vi "Charging_Extract Temp Thresholds From String.vi"(11 "Gen Cals In":string="Reserved[00]=0x00\nReserved[01]=0x00\nReserved[02]=0x00\nReserved[03]=0x00\nReserved[04]=0x00\nReserved[05]=0x00\nReserved[06]=0x00\nReserved[07]=0x00\nReserved[08]=0x00\t\t\nReserved[09]=0x00\nReserved[10]=0x00\nReserved[11]=0x00\nReserved[12]=0x00\nReserved[13]=0x00\nReserved[14]=0x00\ntempMinThreshold=0xCAC4\ntempWarningThresholdl=0x31D3\ntempCriticalThresholdl=0x2FBB\ntempAbortThresholdl=0x2DBD\nthermOffsetMinimum=0x190\nthermOffsetMaximum=0x320\nthermBiasMinimum=0x3E8\nthermBiasMaximum=0xD48\nthermInputMinimum=0x384\nthermInputMaximum=0xC1C\nbatteryIncreasePreCharge=0x19\nbatteryIncreaseConstandCurrent=0x08\nReserved[00]=0x00\nReserved[01]=0x00\nReserved[02]=0x00\nReserved[03]=0x00\nReserved[04]=0x00\nReserved[05]=0x00\nReserved[06]=0x00\nReserved[07]=0x00\nReserved[08]=0x00\nReserved[09]=0x00\nReserved[10]=0x00\nReserved[11]=0x00\nReserved[12]=0x00\nReserved[13]=0x00\nReserved[14]=0x00\nbatteryStateCalStimOff[00]=0xCDE\nbatteryStateCalStimOff[01]=0xC8B\nbatteryStateCalStimOff[02]=0xC4F\nbatteryStateCalStimOff[03]=0xC2E\nbatteryStateCalStimOff[04]=0xC0C\nbatteryStateCalStimOff[05]=0x948\nbatteryStateCalStimOn[00]=0xCCB\nbatteryStateCalStimOn[01]=0xC75\nbatteryStateCalStimOn[02]=0xC3B\nbatteryStateCalStimOn[03]=0xC19\nbatteryStateCalStimOn[04]=0xBFC\nbatteryStateCalStimOn[05]=0x948\nvrectMeasurementCal=0x2EE") -> (0 "Abort Thresholdl (ohms)":dbl=nan format="%.1f", 1 "Critical Thresholdl (ohms)":dbl=nan format="%.1f", 2 "Warning Thresholdl (ohms)":dbl=nan format="%.1f", 3 "Min Threshold (ohms)":dbl=nan format="%.1f")   [LabVIEW 2010]
doc: "This function parses an IPG Temperature Threshold Status string into four Resistance values.\n\nIf the status string format is incorrect, <not available> and NaN values will be returned."
panel:
  # "Temperature thresholds\nin hex multiplied by four."
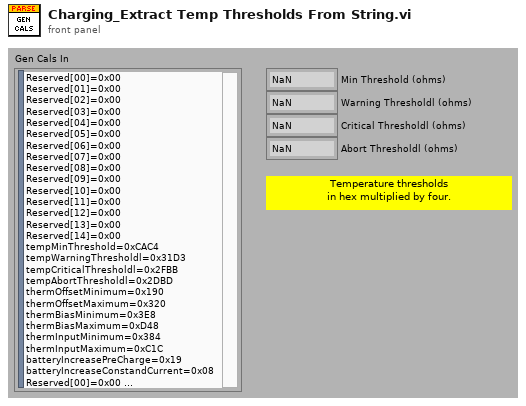
[diagram p1: front panel]
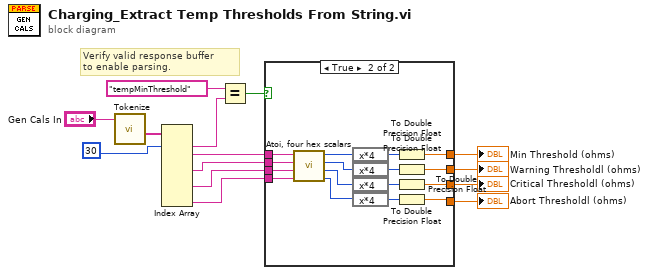
[diagram p0: block diagram]
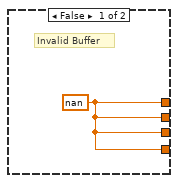
[diagram p2: hidden frame]
diagram:
  # "Verify valid response buffer\nto enable parsing."
  n1 = call "Tokenize.vi"("input string"="Gen Cals In") -> ("tokens"=w13:string[])  [unwired: 4 in, 2 out]
  n2 = Index Array(array=w13, index #1=30 ("index")) -> (element #1=w12:string, element #2=w9:string, element #4=w7:string, element #6=w6:string, element #8=w5:string)  [unwired: 7 in, 3 out]
  n3 = Equal?(x="tempMinThreshold", y=w12) -> (x = y?=w10:bool)
  n4 = case shown="True" w10 {
    tunnel: w9 -> [_ w31]
    tunnel: w7 -> [_ w30]
    tunnel: w6 -> [_ w29]
    tunnel: w5 -> [_ w28]
    tunnel: [w15 w19] -> w4
    tunnel: [w15 w18] -> w3
    tunnel: [w15 w17] -> w2
    tunnel: [w15 w16] -> w1
    frame False {
      w15 = nan
      # "Invalid Buffer"
    }
    frame True {
      n5 = call "Atoi, four hex scalars.vi"("string 4"=w28, "string 3"=w29, "string 2"=w30, "string 1"=w31) -> ("number 4"=w23:i32, "number 3"=w24:i32, "number 2"=w25:i32, "number 1"=w27:i32)  [unwired: 3 in]
      n6 = expression code="x*4"(w27) -> (w26:i32)
      n7 = expression code="x*4"(w25) -> (w22:i32)
      n8 = expression code="x*4"(w24) -> (w21:i32)
      n9 = expression code="x*4"(w23) -> (w20:i32)
      n10 = To Double Precision Float(number=w26) -> (double precision float=w19:dbl)
      n11 = To Double Precision Float(number=w22) -> (double precision float=w18:dbl)
      n12 = To Double Precision Float(number=w21) -> (double precision float=w17:dbl)
      n13 = To Double Precision Float(number=w20) -> (double precision float=w16:dbl)
    }
  }
  "Min Threshold (ohms)" <- w4
  "Warning Thresholdl (ohms)" <- w3
  "Critical Thresholdl (ohms)" <- w2
  "Abort Thresholdl (ohms)" <- w1
